vi "Test All.vi"() -> ()   [LabVIEW 2012]
uses:
  Controls/Wiimote LEDs.ctl
  Controls/Wiimote Buttons.ctl
  Controls/XYZ Acceleration.ctl
  Class/LV Wiimote Interface.lvclass
  <vilib>/picture/3D Picture Control/NI_3D Picture Control.lvlib
panel:
  out "Wiimote LEDs out":T1
  in  "Wiimote Player #":i32=1
  out "# Wiimotes connected":i32
  out "Max Z Accel":sgl
  out "Max Y Accel":sgl
  out "Max X Accel":sgl
  out "BatteryRaw":u8
  out "Tank":sgl(slide) scale=0.0..50.0
  out "Waveform Chart":cluster{"X":sgl, "Y":sgl, "Z":sgl}(graph)
  out "XYZ Acceleration":T2
  out "Wiimote Buttons":T3
  out "error out":errorcluster
  in  "Wiimote LEDs In":T1
  in  "loop rate":u32=100
  in  "stop":bool
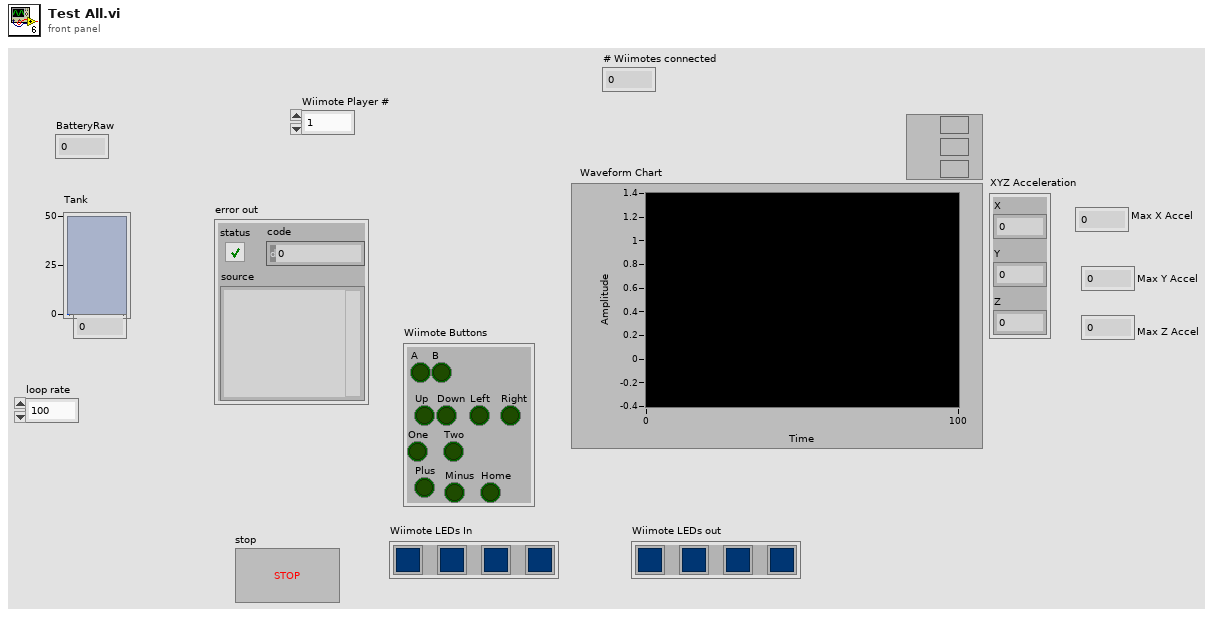
[diagram p1: front panel]
types:
  T1 = typedef "LV Wiimote Interface.lvclass/Wiimote LEDs.ctl" = cluster{"Wiimote LED":bool, "Wiimote LED 2":bool, "Wiimote LED 3":bool, "Wiimote LED 4":bool}
  T2 = typedef "LV Wiimote Interface.lvclass/XYZ Acceleration.ctl" = cluster{"X":sgl, "Y":sgl, "Z":sgl}
  T3 = typedef "LV Wiimote Interface.lvclass/Wiimote Buttons.ctl" = cluster{"A":bool, "B":bool, "Up":bool, "Down":bool, "Left":bool, "Right":bool, "One":bool, "Two":bool, "Plus":bool, "Minus":bool, "Home":bool}
  T4 = typedef "LV Wiimote Interface.ctl" = refnum<class "LV Wiimote Interface.lvclass">
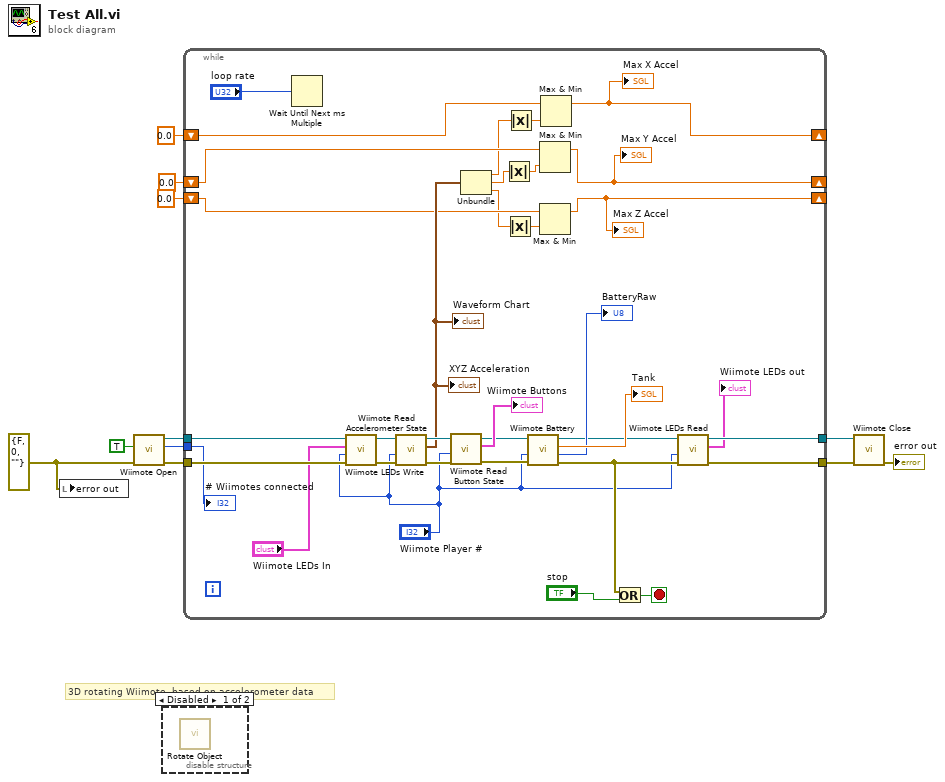
[diagram p0: block diagram]
diagram:
  w5 = errorcluster {"status"=FALSE, "code"=0, "source"=""} ("error out")
  # "3D rotating Wiimote, based on accelerometer data"
  n1 = local write "error out"(w5) -> ()
  n2 = call "Wiimote Open.vi"("error in (no error)"=w5, "Connect to all?"=TRUE) -> ("error out"=w10:errorcluster, "# Wiimotes connected"=w4:i32, "LV WiiMote Interface"=w9:T4)  [unwired: 7 in]
  n3 = disable-structure shown="Disabled" {
    frame Disabled {
      n4 = call <vilib>:"Rotate Object.vi"() -> ()  [unwired: 10 in, 2 out]
    }
    frame Enabled {
    }
  }
  n5 = while {
    tunnel: w10 -> [w44]
    tunnel: w9 -> [w45]
    tunnel: [w15] -> w8
    tunnel: [w14] -> w7
    tunnel: w4 -> [w18]
    shift-right: [w30] -> _
    shift-left: sgl 0.0 ("X") -> [w29]
    shift-right: [w19] -> _
    shift-left: sgl 0.0 ("Y") -> [w28]
    shift-right: [w20] -> _
    shift-left: sgl 0.0 ("Z") -> [w27]
    stop <- w40 stop-if-true
    n6 = Wait Until Next ms Multiple(millisecond multiple="loop rate") -> ()  [unwired: 1 out]
    n7 = call "Wiimote LEDs Write.vi"("error in (no error)"=w44, "Wiimote Player #"="Wiimote Player #", "Wiimote LEDs In"="Wiimote LEDs In", "LV WiiMote Interface In"=w45) -> ("error out"=w38:errorcluster, "LV WiiMote Interface out"=w39:T4)  [unwired: 5 in, 1 out]
    n8 = call "Wiimote Read Accelerometer State.vi"("error in (no error)"=w38, "Wiimote Player #"="Wiimote Player #", "LV WiiMote Interface In"=w39) -> ("error out"=w37:errorcluster, "XYZ Acceleration"=w31:T2, "LV WiiMote Interface out"=w36:T4)  [unwired: 6 in]
    "XYZ Acceleration" <- w31
    "Waveform Chart" <- w31
    n9 = call "Wiimote Read Button State.vi"("error in (no error)"=w37, "Wiimote Player #"="Wiimote Player #", "LV WiiMote Interface In"=w36) -> ("error out"=w34:errorcluster, "Wiimote Buttons"=→"Wiimote Buttons":T3, "LV WiiMote Interface out"=w35:T4)  [unwired: 6 in]
    n10 = Unbundle(w31) -> ("X"=w26:sgl, "Y"=w23:sgl, "Z"=w22:sgl)
    n11 = Absolute Value(x=w23) -> (abs(x)=w24:sgl)
    n12 = Absolute Value(x=w22) -> (abs(x)=w21:sgl)
    n13 = Absolute Value(x=w26) -> (abs(x)=w25:sgl)
    n14 = call "Wiimote Battery.vi"("error in (no error)"=w34, "Wiimote Player #"="Wiimote Player #", "LV WiiMote Interface In"=w35) -> ("error out"=w16:errorcluster, "BatteryRaw"=→"BatteryRaw":u8, "Battery"=→"Tank":sgl, "LV WiiMote Interface out"=w17:T4)  [unwired: 5 in]
    n15 = Max & Min(x=w28, y=w24) -> (max(x,y)=w19:sgl)  [unwired: 1 out]
    "Max Y Accel" <- w19
    n16 = Max & Min(x=w27, y=w21) -> (max(x,y)=w20:sgl)  [unwired: 1 out]
    "Max Z Accel" <- w20
    n17 = Max & Min(x=w29, y=w25) -> (max(x,y)=w30:sgl)  [unwired: 1 out]
    "Max X Accel" <- w30
    n18 = Or(x=w16, y="stop") -> (x .or. y?=w40:bool)
    n19 = call "Wiimote LEDs Read.vi"("error in (no error)"=w16, "Wiimote Player #"="Wiimote Player #", "LV WiiMote Interface In"=w17) -> ("error out"=w14:errorcluster, "Wiimote LEDs out"=→"Wiimote LEDs out":T1, "LV WiiMote Interface out"=w15:T4)  [unwired: 6 in]
    "# Wiimotes connected" <- w18
  }
  n20 = call "Wiimote Close.vi"("error in (no error)"=w7, "LV WiiMote Interface"=w8) -> ("error out"=→"error out":errorcluster)  [unwired: 9 in]
